vi "Stop Core.vi"(10 "final error code":i32, 11 "Sample in":refnum<class "Sample.lvclass">) -> (3 "Sample out":refnum<class "Sample.lvclass">)   [LabVIEW 2022 SP3, in "Sample.lvlib" / "Sample.lvclass"]
doc: "(<B>Filename</B>: Actor Framework.lvlib:Actor.lvclass:Stop Core.vi)\n\nDefines what the actor does before it stops. Use the <B>final error code</B> input to determine whether the actor shut down in response to an error.\n\nBy default, this method does nothing. A descendant class may override it to define behavior, such as shutting down any processes the actor initiated in its override of the Actor Core method."
uses:
  Sample.lvclass
  <vilib>/event_ctls.llb/usereventprio.ctl
  Sample.lvclass/Sample.ctl
  <vilib>/MGI/Monitored Actor/Monitored Actor/Monitored Actor/Monitored Actor.lvclass
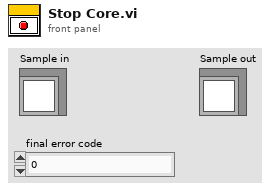
[diagram p1: front panel]
types:
  T1 = typedef "usereventprio.ctl" = enum32{"high priority", "normal priority"}
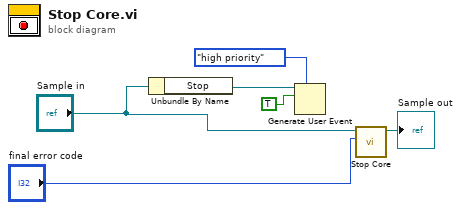
[diagram p0: block diagram]
diagram:
  n1 = Unbundle By Name("Sample in") -> ("Stop"=w2:refnum<user-event>)
  n2 = Generate User Event(priority (normal)=usereventprio."high priority", user event=w2, event data cluster=TRUE ("event data")) -> ()  [unwired: 1 in, 2 out]
  n3 = call-parent "Stop Core.vi"("final error code"="final error code", "Monitored Actor in"="Sample in") -> ("Monitored Actor out"=→"Sample out":refnum<class "Sample.lvclass">)  [unwired: 9 in]
